vi "Scaled Window for 1 Chan (CDB).vi"(8 "error in (no error)":errorcluster, 9 "window parameter":dbl=nan, 10 "window":T1 items=["Rectangle"=0, "Hanning"=1, "Hamming"=2, "Blackman-Harris"=3, "Exact Blackman"=4, "Blackman"=5, "Flat Top"=6, "4 Term B-Harris "=7, "7 Term B-Harris"=8, "Low Sidelobe"=9, "Blackman Nuttall"=11, "Triangle"=30, "Bartlett-Hanning"=31, "Bohman"=32, "Parzen"=33, "Welch"=34, "Kaiser"=60, "Dolph-Chebyshev"=61, "Gaussian"=62], 11 "signal in":waveform(cdb)) -> (0 "error out":errorcluster, 2 "window constants":cluster{"eq noise BW":dbl, "coherent gain":dbl} {"coherent gain" format="%.6f"; "eq noise BW" format="%.6f"}, 3 "signal out":waveform(cdb))   [LabVIEW 2020, in "NI_MAPro.lvlib"]
doc: "Applies a scaled window to the time-domain signal and outputs window constants for further analysis. Wire data to the <B>signal in</B> input to determine the polymorphic instance to use or manually select the instance."
uses:
  NI_MAPro.lvlib
  windowTd.ctl
  NI_MABase.lvlib
  NI_AALPro.lvlib
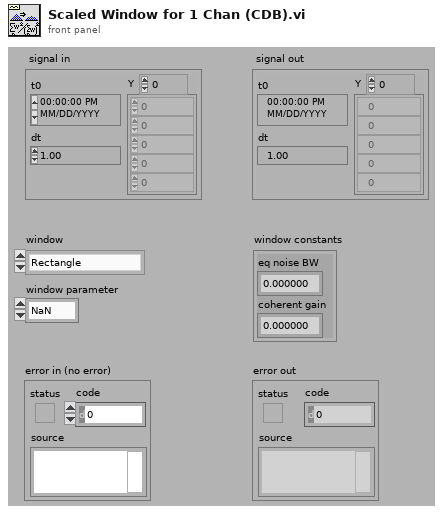
[diagram p1: front panel]
types:
  T1 = typedef "NI_AALPro.lvlib/windowTd.ctl" = u32
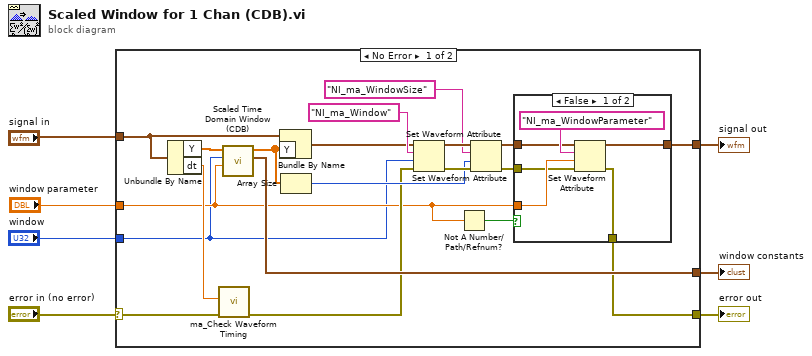
[diagram p0: block diagram]
diagram:
  n1 = case shown="No Error" "error in (no error)" {
    selector: "error in (no error)" -> [w24 w36]
    tunnel: "window" -> [w8 w37]
    tunnel: [w27 w38] -> w7
    tunnel: [w13 w39] -> w5
    tunnel: "signal in" -> [w26 w39]
    tunnel: [w11 w36] -> w2
    tunnel: "window parameter" -> [w10 _]
    frame No Error {
      n2 = Unbundle By Name(w26) -> ("Y"=w25:cdb[], "dt"=w23:dbl)
      n3 = call "ma_Check Waveform Timing.vi"("error in (no error)"=w24, "dt"=w23) -> ("error out"=w12:errorcluster)  [unwired: 8 in, 1 out]
      n4 = call "Scaled Time Domain Window (CDB).vi"("window parameter"=w10, "window"=w8, "X"=w25) -> ("window properties"=w27:cluster{"eq noise BW":dbl, "coherent gain":dbl}, "Windowed X"=w9:cdb[])  [unwired: 6 in, 1 out]
      n5 = Bundle By Name(cluster=w26, "Y"=w9) -> (w14:waveform(cdb))
      n6 = Array Size(array=w9) -> (size(s)=w18:i32)
      n7 = Set Waveform Attribute(4:w12, 5:w8, 6:"NI_ma_Window" ("name"), 7:w14) -> (0:w19:errorcluster, 3:w22:waveform(cdb))  [unwired: 1 out]
      n8 = Not A Number/Path/Refnum?(number/path/refnum=w10) -> (NaN/Path/Refnum?=w15:bool)
      n9 = Set Waveform Attribute(4:w19, 5:w18, 6:"NI_ma_WindowSize" ("name"), 7:w22) -> (0:w16:errorcluster, 3:w17:waveform(cdb))  [unwired: 1 out]
      n10 = case shown="False" w15 {
        tunnel: w17 -> [w32 w35]
        tunnel: [w31 w35] -> w13
        tunnel: w10 -> [w30 _]
        tunnel: [w29 w34] -> w11
        tunnel: w16 -> [w28 w34]
        frame False {
          n11 = Set Waveform Attribute(4:w28, 5:w30, 6:"NI_ma_WindowParameter" ("name"), 7:w32) -> (0:w29:errorcluster, 3:w31:waveform(cdb))  [unwired: 1 out]
        }
        frame True {
        }
      }
    }
    frame Error {
      n12 = call "Scaled Time Domain Window (DBL).vi"("window"=w37) -> ("window properties"=w38:cluster{"eq noise BW":dbl, "coherent gain":dbl})  [unwired: 8 in, 2 out]
    }
  }
  "window constants" <- w7
  "error out" <- w2
  "signal out" <- w5
